vi "Swerve Drive.vi"(1 "Drive Dev Ref":T1[](array[typedef]), 2 "Swerve Dev Ref":T1[](array[typedef]), 4 "X Drive":bool, 5 "error in":errorcluster, 6 "Low Sensitivity":bool, 7 "Z":dbl format="%#_13g", 8 "Reverse Drive":bool, 9 "Straight Drive":bool, 10 "Y":dbl format="%#_13g", 11 "X":dbl format="%#_13g") -> (3 "error out":errorcluster)   [LabVIEW 2017, in "Huskie Swerve.lvlib"]
uses:
  Huskie Swerve.lvlib
  <vilib>/Rock Robotics/WPI/MotorControl/WPI_MotorControlDeviceRef.ctl
  <vilib>/Rock Robotics/WPI/MotorControl/WPI_MotorControlType.ctl
  <vilib>/Rock Robotics/SystemInterfaces/DIO/FPGA_DIOPWMChannel.ctl
  <vilib>/Rock Robotics/WPI/PWM/WPI_PWMDeadband.ctl
  <vilib>/Rock Robotics/SystemInterfaces/DIO/FPGA_DIOChannel.ctl
panel:
  out "Constants":cluster{"a":dbl, "b":dbl, "c":dbl, "d":dbl}[](array[cluster])
  out "Direction":dbl[](array[numeric])
  out "current pos":dbl[](array[numeric])
  out "setpoint":dbl[](array[numeric])
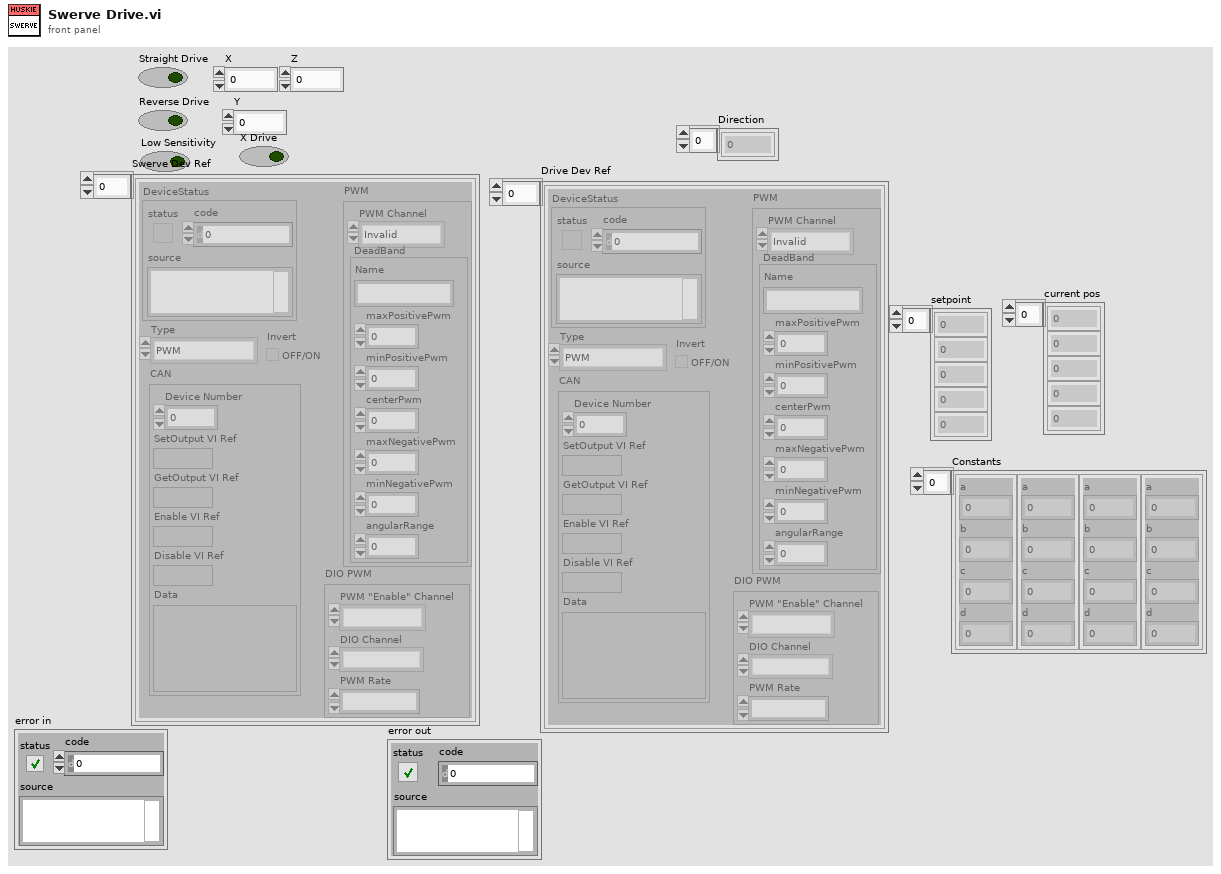
[diagram p1: front panel]
types:
  T1 = typedef "WPI_MotorControlDeviceRef.ctl" = cluster{"DeviceStatus":errorcluster, "Type":T2, "PWM":cluster{"PWM Channel":T3, "DeadBand":T4}, "CAN":cluster{"Device Number":u8, "SetOutput VI Ref":variant, "GetOutput VI Ref":variant, "Enable VI Ref":variant, "Disable VI Ref":variant, "Data":variant}, "Invert":bool, "DIO PWM":cluster{"PWM \"Enable\" Channel":T3, "DIOChannel":T5, "PWM Rate":dbl}}
  T2 = typedef "WPI_MotorControlType.ctl" = enum16{"PWM", "CAN", "DIO PWM"}
  T3 = typedef "FPGA_DIOPWMChannel.ctl" = enum8{"PWM 0", "PWM 1", "PWM 2", "PWM 3", "PWM 4", "PWM 5", "PWM 6", "PWM 7", "PWM 8", "PWM 9", "PWM MXP 0", "PWM MXP 1", "PWM MXP 2", "PWM MXP 3", "PWM MXP 4", "PWM MXP 5", "PWM MXP 6", "PWM MXP 7", "PWM MXP 8", "PWM MXP 9", "Invalid"}
  T4 = typedef "WPI_PWMDeadband.ctl" = cluster{"Name":string, "maxPositivePwm":i32, "minPositivePwm":i32, "centerPwm":i32, "maxNegativePwm":i32, "minNegativePwm":i32, "angularRange":u16}
  T5 = typedef "FPGA_DIOChannel.ctl" = enum8{"DIO 0", "DIO 1", "DIO 2", "DIO 3", "DIO 4", "DIO 5", "DIO 6", "DIO 7", "DIO 8", "DIO 9", "DIO MXP 0", "DIO MXP 1", "DIO MXP 2", "DIO MXP 3", "DIO MXP 4", "DIO MXP 5", "DIO MXP 6", "DIO MXP 7", "DIO MXP 8", "DIO MXP 9", "DIO MXP 10", "DIO MXP 11", "DIO MXP 12", "DIO MXP 13", "DIO MXP 14", "DIO MXP 15", "SPI Port CS1", "SPI Port CS2", "SPI Port CS3", "SPI Port MISO", "SPI Port MOSI", "Invalid"}
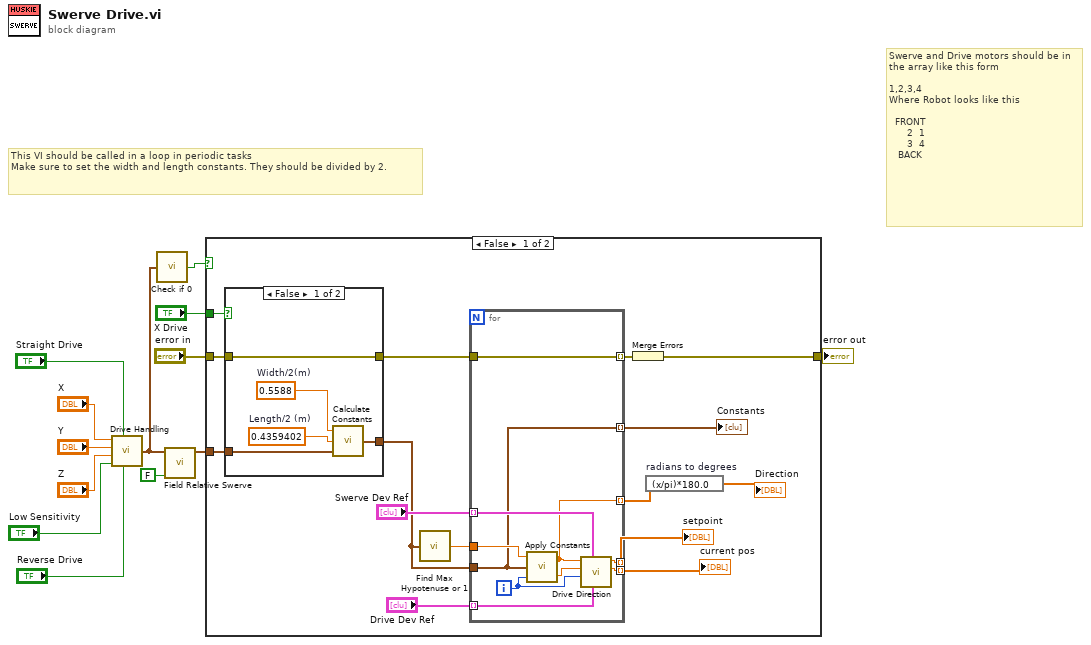
[diagram p0: block diagram]
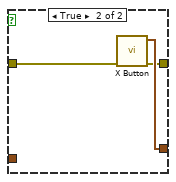
[diagram p2: hidden frame]
diagram:
  # "Swerve and Drive motors should be in the array like this form\n\n1,2,3,4\nWhere Robot looks like this\n\n  FRONT      \n      2  1\n      3  4\n   BACK"
  # "This VI should be called in a loop in periodic tasks\nMake sure to set the width and length constants. They should be divided by 2."
  n1 = call "Drive Handling.vi"("Reverse"="Reverse Drive", "Straight"="Straight Drive", "Low Sensitivity"="Low Sensitivity", "Z"="Z", "Y"="Y", "X"="X") -> ("Axes Magnitudes"=w7:cluster{"X":dbl, "Y":dbl, "Z":dbl})
  n2 = call "Check if 0.vi"("Axes Magnitudes"=w7) -> ("result"=w6:bool)
  n3 = call "Field Relative Swerve.vi"("Field Relative Active"=FALSE, "Axes Magnitudes"=w7) -> ("Axes Mag. Changed"=w2:cluster{"X":dbl, "Y":dbl, "Z":dbl})  [unwired: 9 in]
  n4 = case shown="False" w6 {
    tunnel: w2 -> [w28 _]
    tunnel: "error in" -> [w20 w47]
    tunnel: [w25 w47] -> w4
    tunnel: "X Drive" -> [w21 _]
    frame False {
      n5 = case shown="False" w21 {
        tunnel: w28 -> [w33 _]
        tunnel: [w31 w36] -> w24
        tunnel: w20 -> [w30 w35]
        tunnel: [w30 w34] -> w19
        frame False {
          w29 = 0.4359402  # Length/2 (m)
          w32 = 0.5588  # Width/2(m)
          n6 = call "Calculate Constants.vi"("Axes Magnitudes"=w33, "Length/2"=w29, "Width/2"=w32) -> ("constants cluster"=w31:cluster{"a":dbl, "b":dbl, "c":dbl, "d":dbl})
        }
        frame True {
          n7 = call "X Button.vi"("error in"=w35) -> ("error out"=w34:errorcluster, "constants cluster"=w36:cluster{"a":dbl, "b":dbl, "c":dbl, "d":dbl})  [unwired: 9 in]
        }
      }
      n8 = call "Find Max Hypotenuse or 1.vi"("constants"=w24) -> ("Max or 1"=w23:dbl)
      n9 = for {
        tunnel: w24 -> [w37]
        tunnel: w23 -> [w46]
        tunnel: "Swerve Dev Ref" -> [w44] mode=indexing
        tunnel: "Drive Dev Ref" -> [w43] mode=indexing
        tunnel: [w42] -> w22 mode=indexing
        tunnel: w19 -> [w42]
        tunnel: [w40] -> w18 mode=indexing
        tunnel: [w39] -> w17 mode=indexing
        tunnel: [w38] -> w16 mode=indexing
        tunnel: [w37] -> w14 mode=indexing
        i -> [w41]
        n10 = call "Apply Constants.vi"("Module Number"=w41, "constants cluster"=w37, "Max Speed or 1"=w46) -> ("Magnitude"=w45:dbl, "Desired Direction (rad)"=w38:dbl)
        n11 = call "Drive Direction.vi"("Drive DevRef"=w43, "Swerve DevRef"=w44, "Module Number"=w41, "Wheel Power"=w45, "Desired direction (radians)"=w38) -> ("Sensor Position"=w39:dbl, "setpoint"=w40:dbl)  [unwired: 5 in]
      }
      "setpoint" <- w18
      "current pos" <- w17
      "Constants" <- w14
      n12 = Merge Errors(w22) -> (w25:errorcluster)
      n13 = expression code="(x/pi)*180.0" "radians to degrees"(w16) -> (→"Direction":dbl[])
    }
    frame True {
    }
  }
  "error out" <- w4
